vi "buildClassIcon.vi"(8 "error in (no error)":errorcluster, 10 "className":string, 11 "classPath":path) -> (0 "error out":errorcluster, 3 "classPath(dup)":path)   [LabVIEW 2023]
uses:
  <vilib>/LabVIEW Icon API/lv_icon/Classes/Icon/Icon.lvclass
  <vilib>/LabVIEW Icon API/API_Rectangle Colors.ctl
  <vilib>/LabVIEW Icon API/API_Text.ctl
  <vilib>/LabVIEW Icon API/LabVIEW Icon API.lvlib
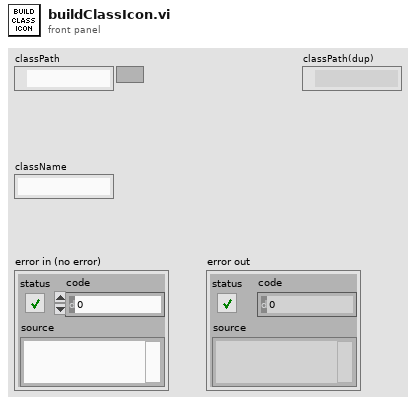
[diagram p1: front panel]
types:
  T1 = typedef "LabVIEW Icon API.lvlib/API_Text.ctl" = cluster{"Line 1 text":string, "Line 2 text":string, "Line 3 text":string, "Line 4 text":string}
  T2 = typedef "LabVIEW Icon API.lvlib/API_Rectangle Colors.ctl" = cluster{"Border":u32, "Background":u32}
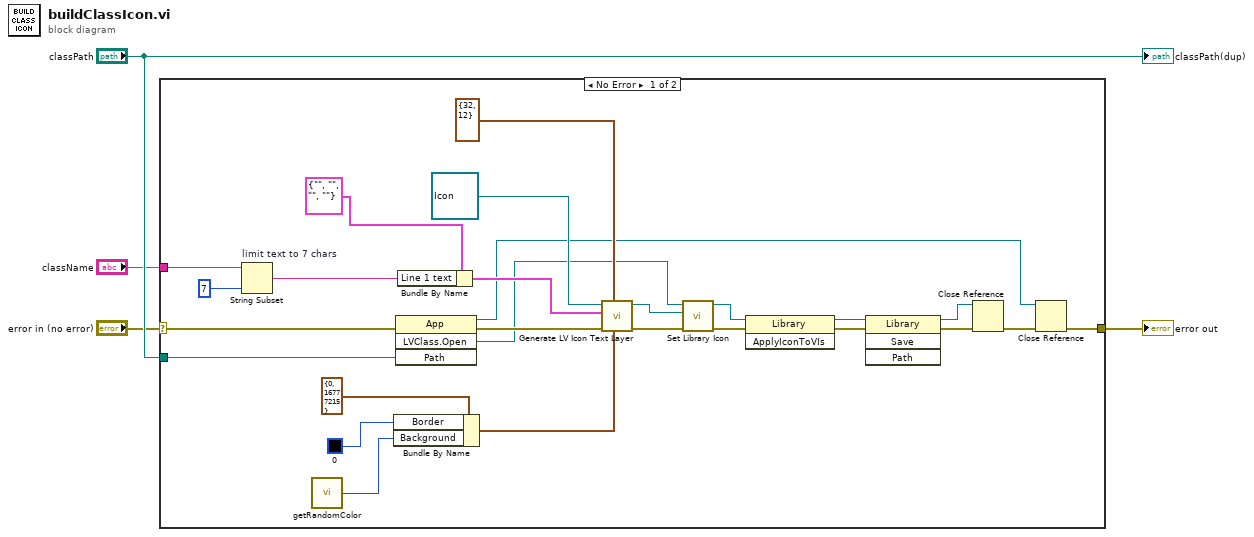
[diagram p0: block diagram]
diagram:
  n1 = case shown="No Error" "error in (no error)" {
    selector: "error in (no error)" -> [w15 w31]
    tunnel: "classPath" -> [w16 _]
    tunnel: [w10 w31] -> w2
    tunnel: "className" -> [w6 _]
    frame No Error {
      n2 = String Subset "limit text to 7 chars"(string=w6, length (rest)=7 ("length (rest)")) -> (substring=w5:string)  [unwired: 1 in]
      n3 = call "getRandomColor.vi"() -> ("color"=w19:u32)
      n4 = Bundle By Name(cluster=T2 {"Border"=0, "Background"=16777215} ("Rectangle colors (black, white)"), "Border"=u32 0 ("Background"), "Background"=w19) -> (w18:T2)
      n5 = invoke class="App" method="LVClass.Open"(error in=w15, "Path"=w16) -> (reference out=w12:refnum<vi>, error out=w14:errorcluster, "LVClass.Open"=w9:refnum<vi>)  [unwired: 2 in, 1 out]
      n6 = Bundle By Name(cluster=T1 {"Line 1 text"="", "Line 2 text"="", "Line 3 text"="", "Line 4 text"=""} ("Text"), "Line 1 text"=w5) -> (w26:T1)
      n7 = call <vilib>:"Generate LV Icon Text Layer.vi"("Rectangle colors (black, white)"=w18, "Rectangle dimension (32,32)"=cluster{"Width":i16, "Height":i16} {"Width"=32, "Height"=12}, "error in (no error)"=w14, "Text"=w26, "Icon in"=refnum<class "Icon.lvclass"> refnum ("Icon.lvclass in")) -> ("error out"=w25:errorcluster, "Icon out"=w27:refnum<class "Icon.lvclass">)  [unwired: 5 in]
      n8 = call <vilib>:"Set Library Icon.vi"("error in (no error)"=w25, "Icon"=w27, "Library Refnum in"=w9) -> ("error out"=w24:errorcluster, "Library Refnum out"=w21:refnum<vi>)  [unwired: 7 in]
      n9 = invoke class="Library" method="ApplyIconToVIs"(reference=w21, error in=w24) -> (reference out=w20:refnum<vi>, error out=w22:errorcluster)  [unwired: 1 in, 1 out]
      n10 = invoke class="Library" method="Save"(reference=w20, error in=w22) -> (reference out=w8:refnum<vi>, error out=w11:errorcluster)  [unwired: 2 in, 2 out]
      n11 = Close Reference(reference=w8, error in (no error)=w11) -> (error out=w13:errorcluster)
      n12 = Close Reference(reference=w12, error in (no error)=w13) -> (error out=w10:errorcluster)
    }
    frame Error {
    }
  }
  "error out" <- w2
  "classPath(dup)" <- "classPath"
